vi "File Path Generation.vi"(7 "Format String":string=".csv", 10 "error in (no error)":errorcluster, 11 "File Path":path=path "C:/data/tdms 5min/tdms 5mintdms 5min.tdms") -> (2 "error out":errorcluster, 3 "appended path":path)   [LabVIEW 2025]
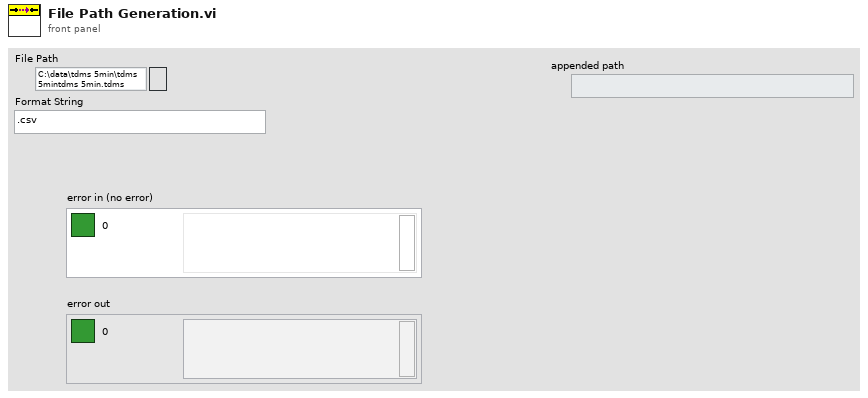
[diagram p1: front panel]
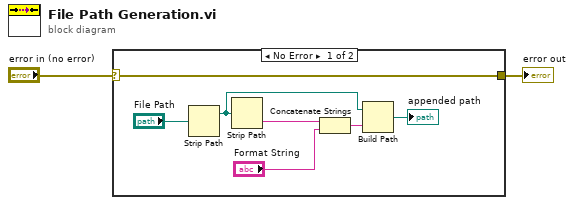
[diagram p0: block diagram]
diagram:
  n1 = case shown="No Error" "error in (no error)" {
    selector: "error in (no error)" -> [w4 _]
    tunnel: [w4 _] -> w1
    frame No Error {
      n2 = Strip Path(path="File Path") -> (stripped path=w8:path)  [unwired: 1 out]
      n3 = Strip Path(path=w8) -> (name=w3:string)  [unwired: 1 out]
      n4 = Concatenate Strings(w3, "Format String") -> (w6:string)
      n5 = Build Path(base path=w8, name or relative path=w6) -> (appended path=→"appended path":path)
    }
    frame Error {
    }
  }
  "error out" <- w1
